vi "Dresser DXD Temp and Press Read Example.vi"(0 "VISA session":refnum<visa-resource-name>, 5 "DXD Address (1)":i32=1 min=1 max=99 step=1, 11 "Error In (no error)":errorcluster) -> (4 "dup VISA session":refnum<visa-resource-name>, 6 "Current Pressure (PSI)":dbl min=-999999.0 max=999999.0 step=1e-05 format="%.3f", 8 "Current Temperature (°C)":dbl min=-999999.0 max=999999.0 step=1e-05 format="%.3f", 15 "Error Out":errorcluster)   [LabVIEW 2010]
doc: "This application example VI demonstrates how to retrieve a pressure reading and then a temperature reading from the Dresser DXD Series pressure transducer at the specified address. The initialize and close VI's need to be added to make this VI usable - See Dresser DXD Temp and Press Read Continuous.vi\n\nWritten by:\nBLOOMY CONTROLS, INC\nWINDSOR, CT 06095, USA\n860-298-9925\nwww.bloomy.com\nV2.0.0\nMay, 2002"
panel:
  # "For instructions on the use of this VI, press Ctrl+H to display the help window and move the mouse over the icon, controls, and indicators"
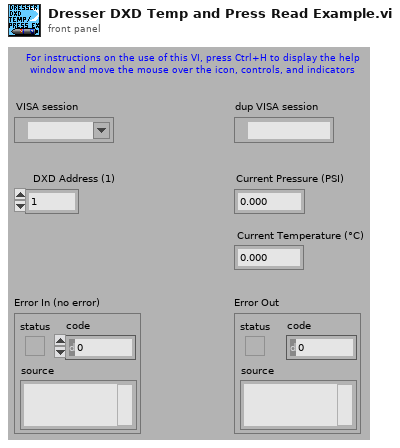
[diagram p1: front panel]
types:
  T1 = enum16{"Error status character set in bit 1 is returned", "No error status character (legacy mode)"}
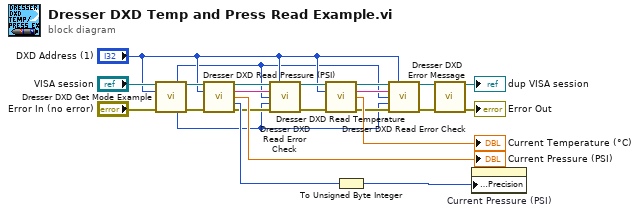
[diagram p0: block diagram]
diagram:
  n1 = call "Dresser DXD Get Mode Example.vi"("VISA session"="VISA session", "DXD Address (1)"="DXD Address (1)", "Error In (no error)"="Error In (no error)") -> ("Bit 1 - Error Status Character"=w2:enum16{"ACK/NAK", "A/N"}, "dup VISA session"=w17:refnum<visa-resource-name>, "Bit 5 - Error Status Character"=w1:T1, "Error Out"=w16:errorcluster)  [unwired: 2 in, 7 out]
  n2 = call "Dresser DXD Read Pressure (PSI).vi"("VISA session"=w17, "DXD Address (1)"="DXD Address (1)", "Error In (no error)"=w16) -> ("dup VISA session"=w12:refnum<visa-resource-name>, "Returned String"=w9:string, "Current Pressure (PSI)"=→"Current Pressure (PSI)":dbl, "Pressure Decimal Position"=w20:i32, "Error Out"=w13:errorcluster)  [unwired: 8 in]
  n3 = call "Dresser DXD Read Error Check.vi"("VISA session"=w12, "DXD Address (1)"="DXD Address (1)", "Returned String (\"\")"=w9, "Mode Bit 1 - Error Status Character"=w2, "Mode Bit 5 - Error Status Character"=w1, "Error In (no error)"=w13) -> ("dup VISA session"=w11:refnum<visa-resource-name>, "Error Out"=w10:errorcluster)  [unwired: 6 in, 2 out]
  n4 = call "Dresser DXD Read Temperature.vi"("VISA session"=w11, "DXD Address (1)"="DXD Address (1)", "Error In (no error)"=w10) -> ("dup VISA session"=w8:refnum<visa-resource-name>, "Returned String"=w3:string, "Current Temperature (°C)"=→"Current Temperature (°C)":dbl, "Error Out"=w7:errorcluster)  [unwired: 9 in]
  n5 = To Unsigned Byte Integer(number=w20) -> (unsigned 8bit integer=w21:u8)
  n6 = call "Dresser DXD Read Error Check.vi"("VISA session"=w8, "DXD Address (1)"="DXD Address (1)", "Returned String (\"\")"=w3, "Mode Bit 1 - Error Status Character"=w2, "Mode Bit 5 - Error Status Character"=w1, "Error In (no error)"=w7) -> ("dup VISA session"=w6:refnum<visa-resource-name>, "Error Out"=w5:errorcluster)  [unwired: 6 in, 2 out]
  n7 = call "Dresser DXD Error Message.vi"("VISA session"=w6, "Error In (no error)"=w5) -> ("dup VISA session"=→"dup VISA session":refnum<visa-resource-name>, "Error Out"=→"Error Out":errorcluster)  [unwired: 9 in, 3 out]
  n8 = property on="Current Pressure (PSI)" class="DigNum (strict)"("Display Format:Precision"=w21) -> ()  [unwired: 2 in, 2 out]
